vi "Constructor.vi"(8 "error in (no error)":errorcluster, 11 "ThickDough in":refnum<class "ThinDough.lvclass">) -> (0 "error out":errorcluster, 2 "Ingredients":string, 3 "ThickDough out":refnum<class "ThinDough.lvclass">)   [LabVIEW 2013, in "ThinDough.lvclass"]
uses:
  ThinDough.lvclass
panel:
  # "我是薄麵皮"
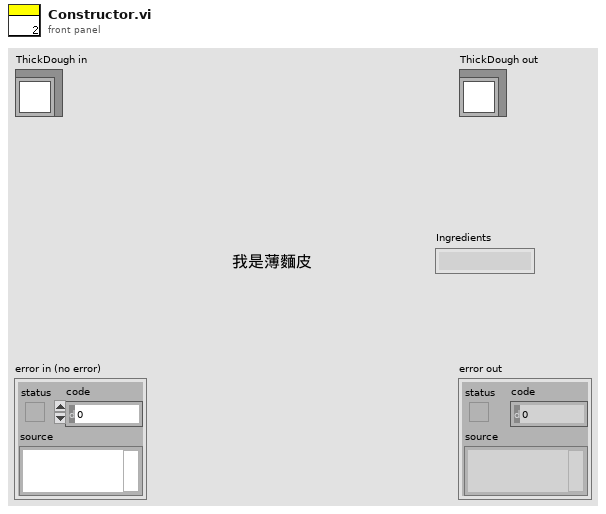
[diagram p1: front panel]
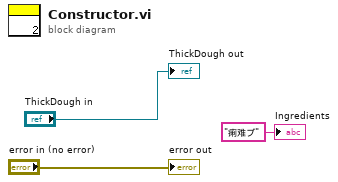
[diagram p0: block diagram]
diagram:
  "error out" <- "error in (no error)"
  "ThickDough out" <- "ThickDough in"
  "Ingredients" <- "痢难ブ" ("Ingredients")
